vi "VA_AO_Init.vi"() -> (0 "error out":errorcluster, 1 "task out":refnum<k21>)   [LabVIEW 2011]
uses:
  <vilib>/DAQmx/create/channels.llb/DAQmx Create Channel (AO-Voltage-Basic).vi
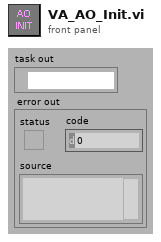
[diagram p1: front panel]
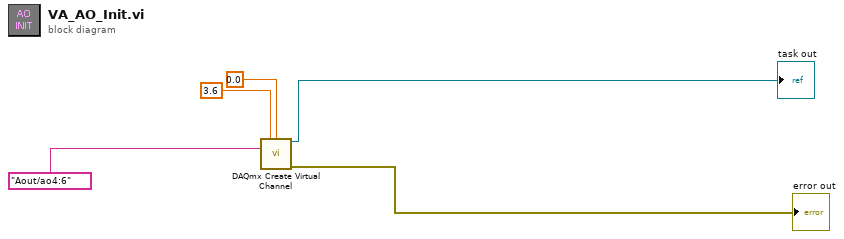
[diagram p0: block diagram]
diagram:
  n1 = call-poly <vilib>:"DAQmx Create Virtual Channel.vi"("maximum value"=3.6 ("Maximum Value Z"), "minimum value"=0.0 ("Minimum Value Z"), "physical channels"=tag "Aout/ao4:6") -> ("task out"=→"task out":refnum<k21>, "error out"=→"error out":errorcluster)  [unwired: 11 in]
